vi "Get VI Parameters and Images.vi"(8 "error in (no error)":errorcluster, 10 "Target Folder":path, 11 "VI Path":path) -> (0 "error out":errorcluster, 1 "Icon Image Path":path, 2 "String":string, 3 "VI Description":string, 5 "VI Name":string, 7 "VI Type":T1(ring))   [LabVIEW 2011]
uses:
  <userlib>/_OpenG.lib/file/file.llb/Strip Path__ogtk.vi
  <userlib>/_OpenG.lib/file/file.llb/Strip Path Extension__ogtk.vi
  <userlib>/_OpenG.lib/file/file.llb/Build Path__ogtk.vi
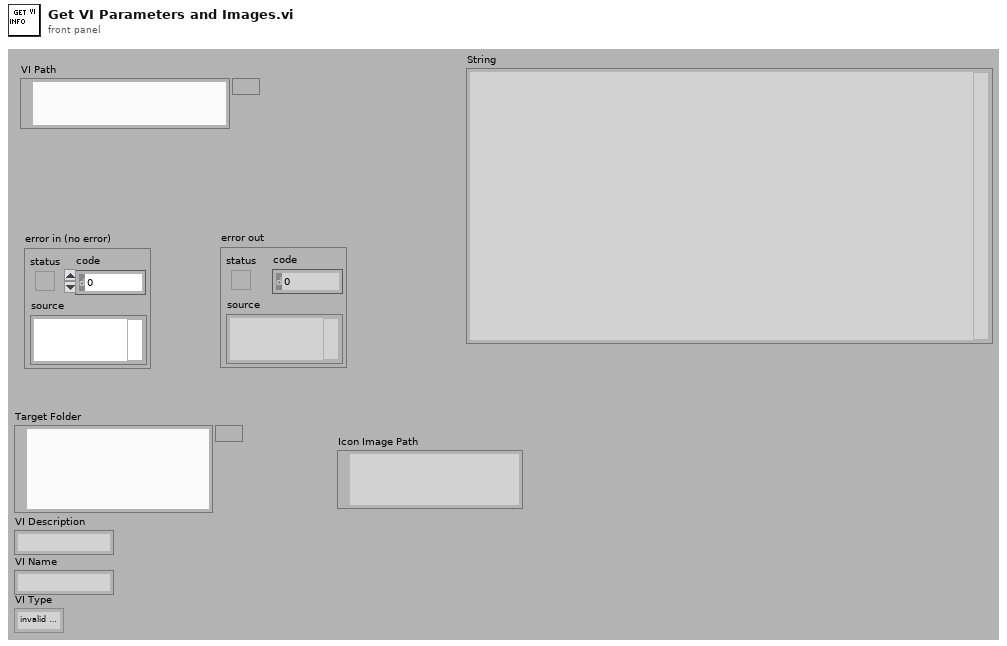
[diagram p1: front panel]
types:
  T1 = enum32{"invalid VI type", "Standard VI", "Control VI", "Global VI", "Polymorphic VI", "Configuration VI"}
  T2 = enum32{"Custom", "Standard", "Using Panel", "Using SubVI", "Complete"}
  T3 = enum32{"invalid VI type", "Standard VI", "Control VI", "Global VI", "Polymorphic VI", "Configuration VI", "SubSystem", "Facade VI", "Method VI", "Statechart Diagram VI"}
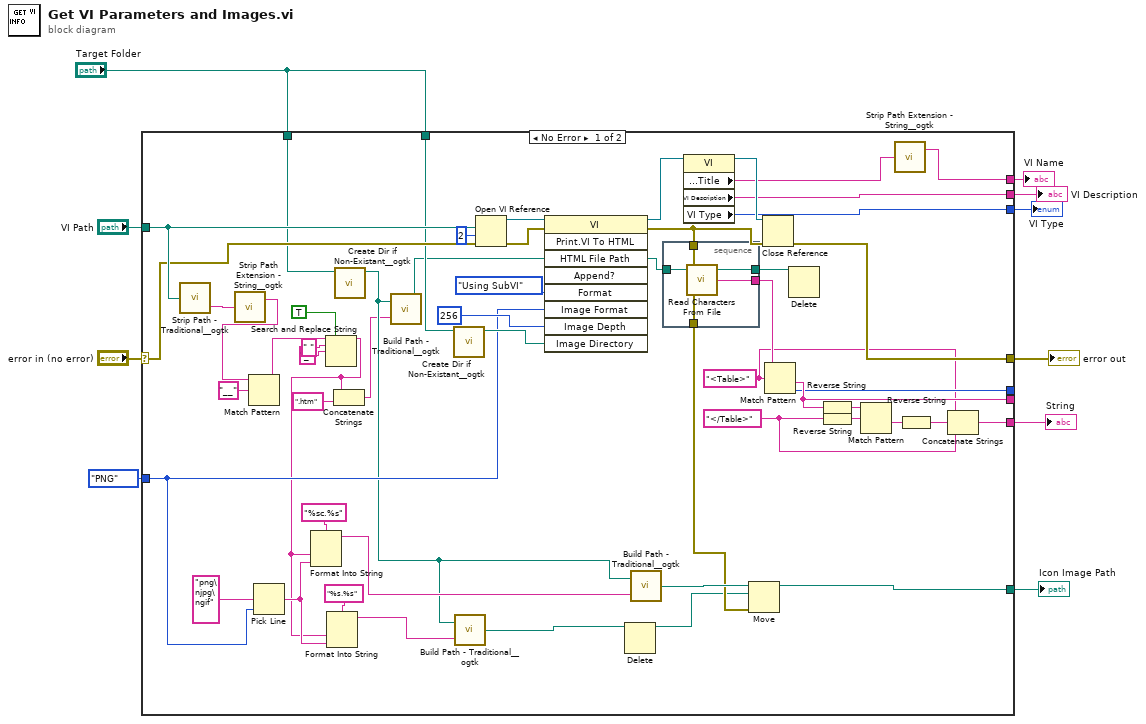
[diagram p0: block diagram]
diagram:
  n1 = case shown="No Error" "error in (no error)" {
    selector: "error in (no error)" -> [w57 w68]
    tunnel: "VI Path" -> [w58 _]
    tunnel: [w55 w68] -> w9
    tunnel: enum32{"PNG", "JPEG", "GIF"}."PNG" ("Image Format") -> [w37 _]
    tunnel: "Target Folder" -> [w54 _]
    tunnel: "Target Folder" -> [w53 _]
    tunnel: [w20 _] -> w6
    tunnel: [w44 _] -> _
    tunnel: [w43 _] -> _
    tunnel: [w24 _] -> w5
    tunnel: [w17 _] -> w3
    tunnel: [w12 _] -> w2
    tunnel: [w11 _] -> w1
    frame No Error {
      w22 = "</Table>" ("regular expression")
      w21 = "<Table>" ("regular expression")
      n2 = call-poly <userlib>:"Strip Path - Traditional__ogtk.vi"("path"=w58) -> ("name"=w15:string)  [unwired: 1 out]
      n3 = call-poly <userlib>:"Strip Path Extension - String__ogtk.vi"("path"=w15) -> ("root"=w16:string)  [unwired: 1 out]
      n4 = Match Pattern(string=w16, regular expression="__") -> (before substring=w27:string)  [unwired: 1 in, 3 out]
      n5 = Pick Line(multi-line string="png\njpg\ngif", line index=w37) -> (output string=w40:string)  [unwired: 1 in]
      n6 = Search and Replace String(replace all?=TRUE ("replace all? (F)"), input string=w27, search string=" ", replace string="_" ("replace string (\"\")")) -> (result string=w25:string)  [unwired: 4 in, 3 out]
      n7 = Format Into String(format string="%sc.%s" ("Format String"), w25, w40) -> (resulting string=w33:string)  [unwired: 2 in, 1 out]
      n8 = Format Into String(format string="%s.%s" ("Format String"), w25, w40) -> (resulting string=w30:string)  [unwired: 2 in, 1 out]
      n9 = Concatenate Strings(w25, ".htm" ("Substring")) -> (w26:string)
      n10 = call <userlib>:"Create Dir if Non-Existant__ogtk.vi"("Directory Path"=w54) -> ("dup Directory Path"=w31:path)  [unwired: 8 in, 2 out]
      n11 = call-poly <userlib>:"Build Path - Traditional__ogtk.vi"("name or relative path"=w26, "base path"=w31) -> ("appended path"=w50:path)
      n12 = call <userlib>:"Create Dir if Non-Existant__ogtk.vi"("Directory Path"=w53) -> ("dup Directory Path"=w52:path)  [unwired: 8 in, 2 out]
      n13 = call-poly <userlib>:"Build Path - Traditional__ogtk.vi"("name or relative path"=w30, "base path"=w31) -> ("appended path"=w29:path)
      n14 = Open VI Reference(vi path=w58, options=2, error in (no error)=w57) -> (vi reference=w60:refnum<vi>, error out=w63:errorcluster)  [unwired: 3 in]
      n15 = invoke class="VI" method="Print.VI To HTML"(reference=w60, error in=w63, "HTML File Path"=w50, "Format"=T2."Using SubVI", "Image Format"=w37, "Image Depth"=256, "Image Directory"=w52) -> (reference out=w19:refnum<vi>, error out=w49:errorcluster)  [unwired: 2 in, 7 out]
      n16 = Delete(path (use dialog)=w29) -> (deleted path=w28:path)  [unwired: 4 in, 2 out]
      n17 = call-poly <userlib>:"Build Path - Traditional__ogtk.vi"("name or relative path"=w33, "base path"=w31) -> ("appended path"=w42:path)
      n18 = stacked-sequence {
        tunnel: w50 -> [w67]
        tunnel: w49 -> [w65]
        tunnel: [w66] -> w48
        tunnel: [w65] -> w38
        tunnel: [w64] -> w14
        frame #0 {
          n19 = call <vilib>:"Read Characters From File.vi"("file path (dialog if empty)"=w67) -> ("new file path (NotAPath if cancelled)"=w64:path, "character string"=w66:string)  [unwired: 5 in, 2 out]
        }
      }
      n20 = property class="VI"(reference=w19) -> (reference out=w18:refnum<vi>, "Front Panel Window:Title"=w13:string, "VI Description"=w17:string, "VI Type"=w11:T3)  [unwired: 1 in, 1 out]
      n21 = Move(source path=w42, error in=w38, 10:w28) -> (3:w24:path)  [unwired: 2 in, 2 out]
      n22 = Close Reference(reference=w18, error in (no error)=w49) -> (error out=w55:errorcluster)
      n23 = Match Pattern(string=w48, regular expression=w21) -> (after substring=w44:string, offset past match=w43:i32)  [unwired: 1 in, 2 out]
      n24 = Delete(path (use dialog)=w14) -> ()  [unwired: 4 in, 3 out]
      n25 = Reverse String(1:w44) -> (0:w47:string)
      n26 = Reverse String(1:w22) -> (0:w46:string)
      n27 = Match Pattern(string=w47, regular expression=w46) -> (after substring=w45:string)  [unwired: 1 in, 3 out]
      n28 = call-poly <userlib>:"Strip Path Extension - String__ogtk.vi"("path"=w13) -> ("root"=w12:string)  [unwired: 1 out]
      n29 = Reverse String(1:w45) -> (0:w23:string)
      n30 = Concatenate Strings(w21, w23, w22) -> (w20:string)
    }
    frame Error {
    }
  }
  "error out" <- w9
  "String" <- w6
  "Icon Image Path" <- w5
  "VI Description" <- w3
  "VI Name" <- w2
  "VI Type" <- w1
